vi "VI Tree.vi"   [LabVIEW 2021, in "Siglent SDS 1000 2000 Series.lvlib"]
doc: "This is the instrument driver for the Siglent SDS 1000 2000 Series Oscilloscopes. The VI Tree displays all the user-callable VIs of the instrument driver in an organized table."
uses:
  <instrlib>/Siglent SDS 1000 2000 Series/Siglent SDS 1000 2000 Series.lvlib
  <instrlib>/Siglent SDS 1000 2000 Series/Public/Data/Read Waveform Measurement (Standard).vi
  <instrlib>/Siglent SDS 1000 2000 Series/Public/Configure/Configure Trigger (Edge).vi
  <instrlib>/Siglent SDS 1000 2000 Series/Public/Data/Read Waveform (Single).vi
panel:
  # "(c) 2015 SIGLENT TECHNOLOGIES CO., LTD.   ALL RIGHTS RESERVED."
  # "SEE DIAGRAM\nFOR VI TREE."
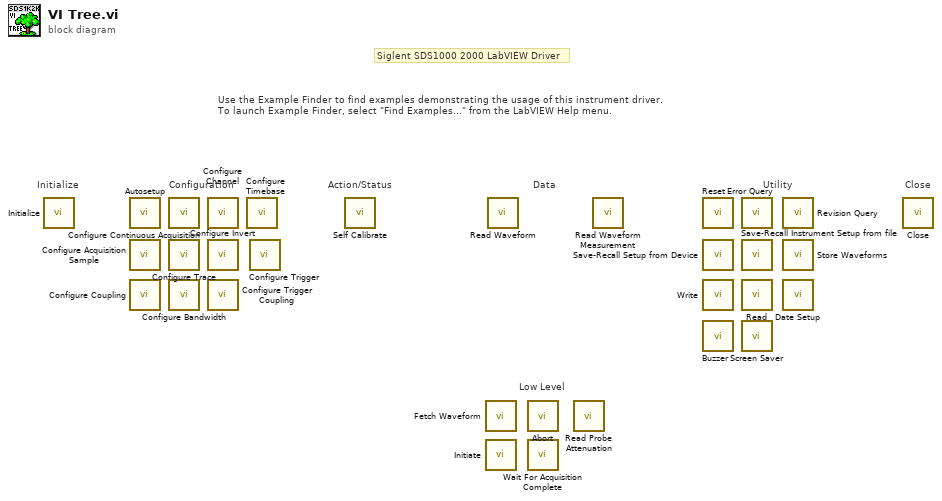
[diagram p0: block diagram]
diagram:
  # "Siglent SDS1000 2000 LabVIEW Driver"
  # "Low Level"
  # "Action/Status"
  # "Use the Example Finder to find examples demonstrating the usage of this instrument driver.\nTo launch Example Finder, select \"Find Examples...\" from the LabVIEW Help menu."
  # "Configuration"
  # "Utility"
  # "Data"
  # "Close"
  # "Initialize"
  n1 = call <instrlib>:"Initialize.vi"() -> ()  [unwired: 10 in, 2 out]
  n2 = call <instrlib>:"Autosetup.vi"() -> ()  [unwired: 10 in, 2 out]
  n3 = call <instrlib>:"Configure Acquisition Sample.vi"() -> ()  [unwired: 10 in, 2 out]
  n4 = call <instrlib>:"Configure Coupling.vi"() -> ()  [unwired: 10 in, 2 out]
  n5 = call <instrlib>:"Configure Continuous Acquisition.vi"() -> ()  [unwired: 10 in, 2 out]
  n6 = call <instrlib>:"Configure Trace.vi"() -> ()  [unwired: 10 in, 2 out]
  n7 = call <instrlib>:"Configure Bandwidth.vi"() -> ()  [unwired: 10 in, 2 out]
  n8 = call <instrlib>:"Configure Channel.vi"() -> ()  [unwired: 14 in, 2 out]
  n9 = call <instrlib>:"Configure Invert.vi"() -> ()  [unwired: 10 in, 2 out]
  n10 = call <instrlib>:"Configure Trigger Coupling.vi"() -> ()  [unwired: 10 in, 2 out]
  n11 = call <instrlib>:"Configure Timebase.vi"() -> ()  [unwired: 10 in, 2 out]
  n12 = call-poly <instrlib>:"Configure Trigger.vi"() -> ()  [unwired: 14 in, 2 out]
  n13 = call <instrlib>:"Self Calibrate.vi"() -> ()  [unwired: 10 in, 2 out]
  n14 = call <instrlib>:"Fetch Waveform.vi"() -> ()  [unwired: 9 in, 3 out]
  n15 = call <instrlib>:"Initiate.vi"() -> ()  [unwired: 10 in, 2 out]
  n16 = call-poly <instrlib>:"Read Waveform.vi"() -> ()  [unwired: 9 in, 3 out]
  n17 = call <instrlib>:"Abort.vi"() -> ()  [unwired: 10 in, 2 out]
  n18 = call <instrlib>:"Wait For Acquisition Complete.vi"() -> ()  [unwired: 9 in, 3 out]
  n19 = call <instrlib>:"Read Probe Attenuation.vi"() -> ()  [unwired: 9 in, 3 out]
  n20 = call-poly <instrlib>:"Read Waveform Measurement.vi"() -> ()  [unwired: 13 in, 3 out]
  n21 = call <instrlib>:"Reset.vi"() -> ()  [unwired: 10 in, 2 out]
  n22 = call <instrlib>:"Save-Recall Setup from Device.vi"() -> ()  [unwired: 10 in, 2 out]
  n23 = call <instrlib>:"Write.vi"() -> ()  [unwired: 9 in, 3 out]
  n24 = call <instrlib>:"Buzzer.vi"() -> ()  [unwired: 10 in, 2 out]
  n25 = call <instrlib>:"Error Query.vi"() -> ()  [unwired: 8 in, 4 out]
  n26 = call <instrlib>:"Save-Recall Instrument Setup from file.vi"() -> ()  [unwired: 14 in, 2 out]
  n27 = call <instrlib>:"Read.vi"() -> ()  [unwired: 8 in, 4 out]
  n28 = call <instrlib>:"Screen Saver.vi"() -> ()  [unwired: 10 in, 2 out]
  n29 = call <instrlib>:"Revision Query.vi"() -> ()  [unwired: 8 in, 4 out]
  n30 = call <instrlib>:"Store Waveforms.vi"() -> ()  [unwired: 10 in, 2 out]
  n31 = call <instrlib>:"Date Setup.vi"() -> ()  [unwired: 14 in, 2 out]
  n32 = call <instrlib>:"Close.vi"() -> ()  [unwired: 11 in, 1 out]
